vi "PopModuleTypes.vi"(8 "ErrorArray In":errorcluster[](array[cluster])) -> (0 "ErrorArray Out":errorcluster[](array[cluster]))   [LabVIEW 2017, in "Framework.lvlib"]
uses:
  Framework.lvlib
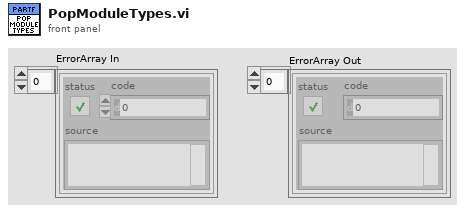
[diagram p1: front panel]
types:
  T1 = typedef "Framework.lvlib/clFrontPanelControlRefs.ctl" = cluster{"TestFilePathRef":refnum<vi>, "BusNumberRef":refnum<vi>, "NumberOfBusesRef":refnum<vi>, "EvtTypeRef":refnum<vi>, "EvtParamsRef":refnum<vi>, "EvtConfigRef":refnum<vi>, "StartTimeRef":refnum<vi>, "EndTimeRef":refnum<vi>, "PmuImpairTypeRef":refnum<vi>, "PmuImpairParamsRef":refnum<vi>, "NetImpairParamsRef":refnum<vi>, "FlagImpairTypeRef":refnum<vi>, "FlagImpairParamsRef":refnum<vi>, "NetImpairTypeRef":refnum<vi>, "OutputFileType":refnum<vi>, "PmuImpairConfigRef":refnum<vi>, "AppTypeRef":refnum<vi>, "ScriptPathRef":refnum<vi>, "ShowPanels?":refnum<vi>}
  T2 = typedef "Framework.lvlib/clFrameworkData.ctl" = cluster{"EvtINIFilePaths":path[], "BusClassInstances":refnum<class "Bus.lvclass">[], "PmuImpairINIFilePaths":path[], "FlagImpairINIFilePaths":path[], "NetImpairINIFilePaths":path[], "OutputToFileINIFilePaths":path[], "AppINIFilePaths":path[], "AppModuleID":i32, "OutputToFileID":i32}
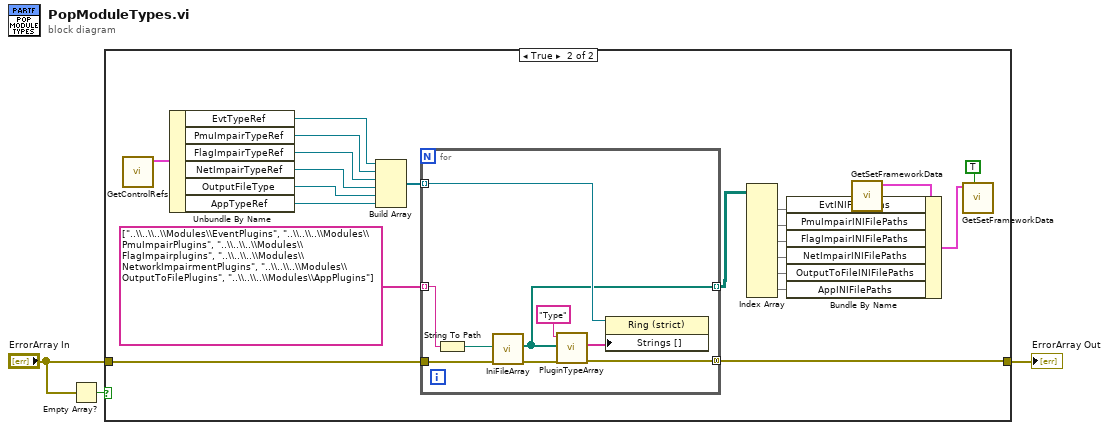
[diagram p0: block diagram]
diagram:
  n1 = Empty Array?(array="ErrorArray In") -> (empty?=w3:bool)
  n2 = case shown="True" w3 {
    tunnel: "ErrorArray In" -> [w4 w16]
    tunnel: [w4 w15] -> w1
    frame False {
    }
    frame True {
      n3 = call "GetControlRefs.vi"() -> ("clControlRefs Out"=w25:T1)  [unwired: 11 in]
      n4 = Unbundle By Name(w25) -> ("EvtTypeRef"=w23:refnum<vi>, "PmuImpairTypeRef"=w22:refnum<vi>, "FlagImpairTypeRef"=w21:refnum<vi>, "NetImpairTypeRef"=w20:refnum<vi>, "OutputFileType"=w19:refnum<vi>, "AppTypeRef"=w18:refnum<vi>)
      n5 = Build Array(w23, w22, w21, w20, w19, w18) -> (w17:refnum<vi>[])
      n6 = for {
        tunnel: string[] ["..\\..\\..\\Modules\\EventPlugins", "..\\..\\..\\Modules\\PmuImpairPlugins", "..\\..\\..\\Modules\\FlagImpairplugins", "..\\..\\..\\Modules\\NetworkImpairmentPlugins", "..\\..\\..\\Modules\\OutputToFilePlugins", "..\\..\\..\\Modules\\AppPlugins"] -> [w34] mode=indexing
        tunnel: w17 -> [w30] mode=indexing
        tunnel: w16 -> [w28]
        tunnel: [w27] -> w15 mode=concatenating
        tunnel: [w26] -> w13 mode=indexing
        n7 = String To Path(string=w34) -> (path=w33:path)
        n8 = call "IniFileArray.vi"("ErrorArray In"=w28, "Relative Path to Plugins"=w33) -> ("ErrorArray Out"=w31:errorcluster[], "INIFilePaths"=w26:path[])  [unwired: 8 in]
        n9 = call "PluginTypeArray.vi"("ErrorArray Out in"=w31, "INIFilePaths"=w26, "section"="Type") -> ("ErrorArray Out out"=w27:errorcluster[], "PluginTypes"=w29:string[])  [unwired: 6 in, 1 out]
        n10 = property class="Ring (strict)"(reference=w30, "Strings []"=w29) -> ()  [unwired: 1 in, 2 out]
      }
      n11 = Index Array(array=w13) -> (element #1=w12:path[], element #2=w11:path[], element #3=w10:path[], element #4=w9:path[], element #5=w8:path[], element #6=w7:path[])  [unwired: 12 in]
      n12 = call "GetSetFrameworkData.vi"() -> ("clFrameworkData Out"=w14:T2)  [unwired: 11 in]
      n13 = Bundle By Name(cluster=w14, "EvtINIFilePaths"=w12, "PmuImpairINIFilePaths"=w11, "FlagImpairINIFilePaths"=w10, "NetImpairINIFilePaths"=w9, "OutputToFileINIFilePaths"=w8, "AppINIFilePaths"=w7) -> (w6:T2)
      n14 = call "GetSetFrameworkData.vi"("Set (F)"=TRUE, "clFrameworkData In"=w6) -> ()  [unwired: 9 in, 1 out]
    }
  }
  "ErrorArray Out" <- w1
